vi "BigIntDevide.vi"(2 "b":cluster{"Boolean":bool, "Array":u64[]}, 3 "a":cluster{"Boolean":bool, "Array":u64[]}) -> (0 "a % b":cluster{"Boolean":bool, "Array":u64[]}, 1 "a / b":cluster{"Boolean":bool, "Array":u64[]})   [LabVIEW 2023]
panel:
  out "|b|":cluster{bool, "Array":u64[]}
  out "|a|":cluster{bool, "Array":u64[]}
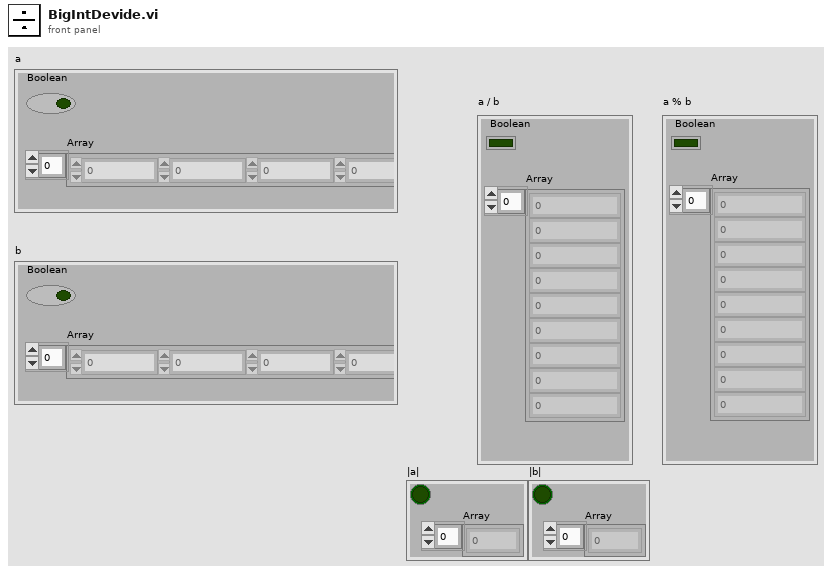
[diagram p1: front panel]
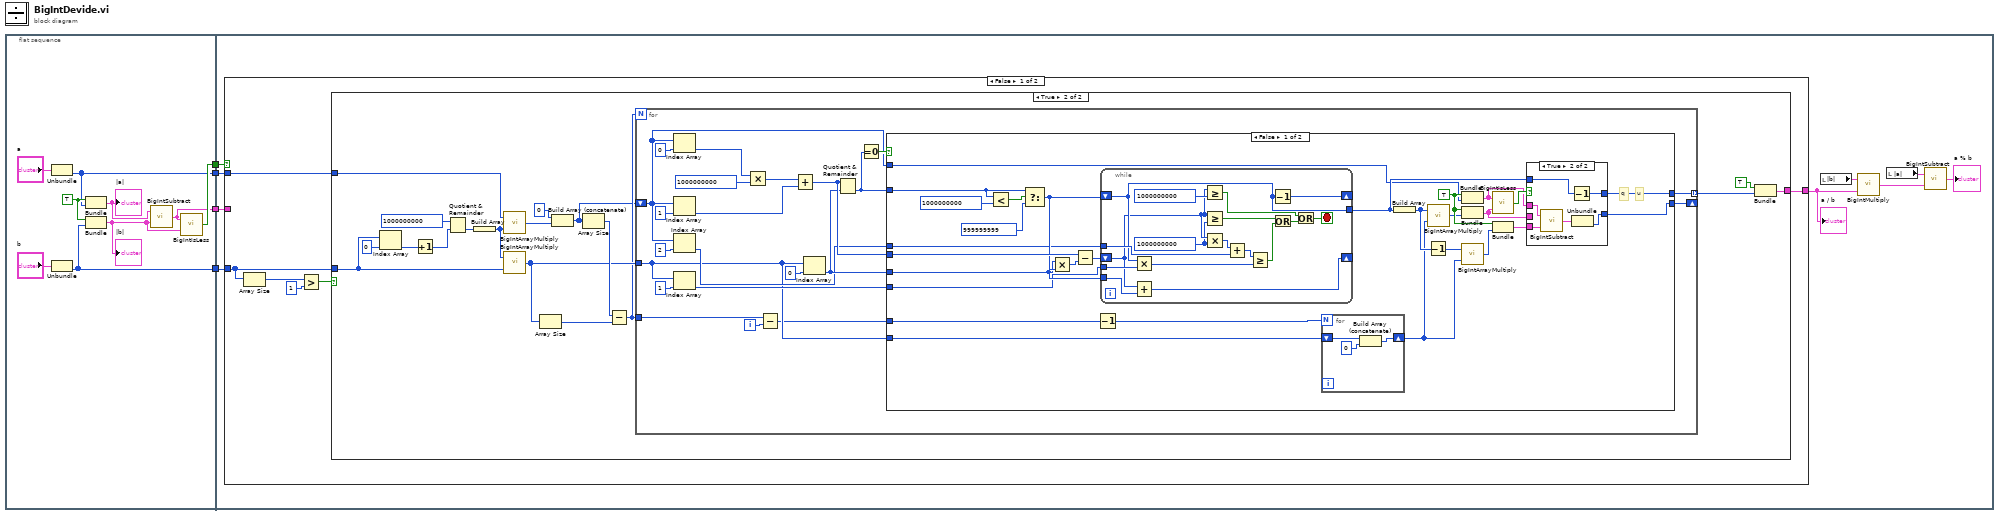
[diagram p0: block diagram]
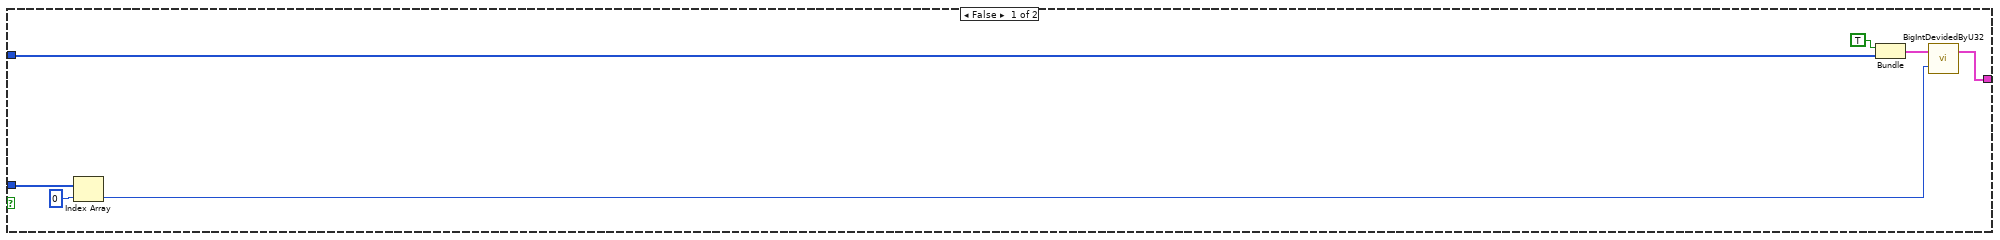
[diagram p2: hidden frame]
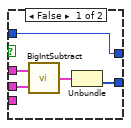
[diagram p3: hidden frame]
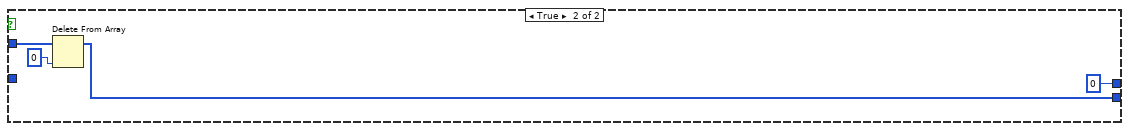
[diagram p4: hidden frame]
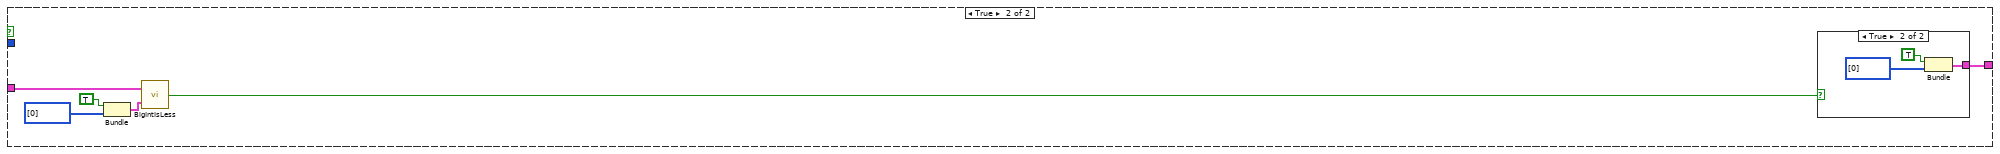
[diagram p5: hidden frame]
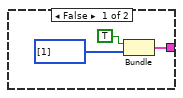
[diagram p6: hidden frame]
diagram:
  n1 = flat-sequence {
    tunnel: [w5] -> w4
    tunnel: [w6] -> w3
    tunnel: [w8] -> w2
    tunnel: [w7] -> w1
    tunnel: w4 -> [w17]
    tunnel: w3 -> [w16]
    tunnel: w2 -> [w15]
    tunnel: w1 -> [w14]
    frame #0 {
      w9 = TRUE
      n2 = Unbundle("a") -> ("Array"=w5:u64[])  [unwired: 1 out]
      n3 = Unbundle("b") -> ("Array"=w6:u64[])  [unwired: 1 out]
      n4 = Bundle(w9, "Array"=w5) -> (w12:cluster{bool, "Array":u64[]})  [unwired: 1 in]
      "|a|" <- w12
      n5 = Bundle(w9, "Array"=w6) -> (w13:cluster{bool, "Array":u64[]})  [unwired: 1 in]
      "|b|" <- w13
      n6 = call "BigIntSubtract.vi"("b"=w13, "a"=w12) -> ("a - b"=w7:cluster{"Boolean":bool, "Array":u64[]})
      n7 = call "BigIntIsLess.vi"("b"=w13, "a"=w7) -> ("a < b"=w8:bool)
    }
    frame #1 {
      n8 = case shown="False" w15 {
        tunnel: [w28 w139] -> w22
        tunnel: w17 -> [w27 _]
        tunnel: w16 -> [w26 _]
        tunnel: w14 -> [_ w142]
        frame False {
          n9 = Array Size(array=w26) -> (size(s)=w25:i32)
          n10 = Greater?(x=w25, y=1) -> (0:w23:bool)
          n11 = case shown="True" w23 {
            tunnel: [w29 w40] -> w28
            tunnel: w27 -> [w34 w39]
            tunnel: w26 -> [w33 w38]
            frame False {
              n12 = Index Array(array=w33, index=0) -> (element=w30:u64)
              n13 = Bundle(TRUE, "Array"=w34) -> (w31:cluster{bool, "Array":u64[]})  [unwired: 1 in]
              n14 = call "BigIntDevidedByU32.vi"("b (<1e9)"=w30, "a"=w31) -> ("a / b"=w29:cluster{"Boolean":bool, "Array":u64[]})  [unwired: 1 out]
            }
            frame True {
              n15 = Index Array(array=w38, index=0) -> (element=w52:u64)
              n16 = Increment(x=w52) -> (x+1=w51:u64)
              n17 = Quotient & Remainder(x=u64 1000000000, y=w51) -> (floor(x/y)=w49:u64)  [unwired: 1 out]
              n18 = Build Array(w49) -> (w48:u64[])
              n19 = call "BigIntArrayMultiply.vi"("b"=w48, "a"=w39) -> ("a * b"=w45:u64[])
              n20 = call "BigIntArrayMultiply.vi"("b"=w38, "a"=w48) -> ("a * b"=w44:u64[])
              n21 = Array Size(array=w44) -> (size(s)=w46:i32)
              n22 = Build Array (concatenate)(u64 0, w45) -> (w37:u64[])
              n23 = Array Size(array=w37) -> (size(s)=w47:i32)
              n24 = Subtract(x=w47, y=w46) -> (x-y=w43:i32)
              n25 = for {
                N: w43 -> [_]
                tunnel: w44 -> [w66]
                shift-right: [w60] -> _
                shift-left: w37 -> [w58]
                tunnel: w43 -> [w63]
                tunnel: [w61] -> w42 mode=indexing
                i -> [w57]
                n26 = Index Array(array=w58, index=0) -> (element=w59:u64)
                n27 = Index Array(array=w58, index=1) -> (element=w74:u64)
                n28 = Index Array(array=w58, index=2) -> (element=w67:u64)
                n29 = Index Array(array=w66, index=1) -> (element=w68:u64)
                n30 = Multiply(x=w59, y=u64 1000000000) -> (x*y=w65:u64)
                n31 = Subtract(x=w63, y=w57) -> (x-y=w62:i32)
                n32 = Add(x=w65, y=w74) -> (x+y=w71:u64)
                n33 = Index Array(array=w66, index=0) -> (element=w70:u64)
                n34 = Quotient & Remainder(x=w71, y=w70) -> (floor(x/y)=w72:u64)  [unwired: 1 out]
                n35 = Equal To 0?(x=w72) -> (x = 0?=w73:bool)
                n36 = case shown="False" w73 {
                  tunnel: w72 -> [w101 _]
                  tunnel: w71 -> [w99 _]
                  tunnel: w70 -> [w95 _]
                  tunnel: w68 -> [w94 _]
                  tunnel: w67 -> [w93 _]
                  tunnel: w58 -> [w83 w138]
                  tunnel: w66 -> [w92 _]
                  tunnel: w62 -> [w91 _]
                  tunnel: [w86 0] -> w61
                  tunnel: [w76 w136] -> w60
                  frame False {
                    w84 = TRUE
                    # "u"
                    # "q"
                    n37 = Less?(x=w101, y=u64 1000000000) -> (x < y?=w102:bool)
                    n38 = Select(t=w101, s=w102, f=u64 999999999) -> (s? t:f=w96:u64)
                    n39 = Multiply(x=w95, y=w96) -> (x*y=w98:u64)
                    n40 = Subtract(x=w99, y=w98) -> (x-y=w97:u64)
                    n41 = Decrement(x=w91) -> (x-1=w85:i32)
                    n42 = while {
                      tunnel: w95 -> [w133]
                      tunnel: w94 -> [w134]
                      shift-right: [w132] -> _
                      shift-left: w97 -> [w122]
                      shift-right: [w131] -> _
                      shift-left: w96 -> [w126]
                      tunnel: w93 -> [w129]
                      tunnel: [w126] -> w87
                      stop <- w123 stop-if-true
                      w121 = u64 1000000000
                      n43 = Multiply(x=w126, y=w134) -> (x*y=w127:u64)
                      n44 = Add(x=w122, y=w133) -> (x+y=w132:u64)
                      n45 = Greater Or Equal?(x=w122, y=u64 1000000000) -> (x >= y?=w124:bool)
                      n46 = Greater Or Equal?(x=w122, y=w121) -> (x >= y?=w120:bool)
                      n47 = Multiply(x=w122, y=w121) -> (x*y=w130:u64)
                      n48 = Add(x=w130, y=w129) -> (x+y=w128:u64)
                      n49 = Greater Or Equal?(x=w128, y=w127) -> (x >= y?=w119:bool)
                      n50 = Decrement(x=w126) -> (x-1=w131:u64)
                      n51 = Or(x=w120, y=w119) -> (x .or. y?=w118:bool)
                      n52 = Or(x=w124, y=w118) -> (x .or. y?=w123:bool)
                    }
                    n53 = for {
                      N: w85 -> [_]
                      shift-right: [w115] -> w89
                      shift-left: w92 -> [w117]
                      n54 = Build Array (concatenate)(w117, u64 0) -> (w115:u64[])
                    }
                    n55 = Build Array(w87) -> (w90:u64[])
                    n56 = Decrement(x=w90) -> (x-1=w88:u64[])
                    n57 = call "BigIntArrayMultiply.vi"("b"=w89, "a"=w90) -> ("a * b"=w82:u64[])
                    n58 = Bundle(w84, w83) -> (w79:cluster{bool, u64[]})  [unwired: 1 in]
                    n59 = Bundle(w84, "a * b"=w82) -> (w78:cluster{bool, "a * b":u64[]})  [unwired: 1 in]
                    n60 = call "BigIntArrayMultiply.vi"("b"=w89, "a"=w88) -> ("a * b"=w81:u64[])
                    n61 = call "BigIntIsLess.vi"("b"=w78, "a"=w79) -> ("a < b"=w80:bool)
                    n62 = Bundle(w84, "a * b"=w81) -> (w77:cluster{bool, "a * b":u64[]})  [unwired: 1 in]
                    n63 = case shown="True" w80 {
                      tunnel: w87 -> [w108 w114]
                      tunnel: [w108 w113] -> w86
                      tunnel: w79 -> [w107 w110]
                      tunnel: w78 -> [w106 _]
                      tunnel: w77 -> [_ w111]
                      tunnel: [w104 w109] -> w76
                      frame False {
                        n64 = call "BigIntSubtract.vi"("b"=w106, "a"=w107) -> ("a - b"=w105:cluster{"Boolean":bool, "Array":u64[]})
                        n65 = Unbundle(w105) -> ("Array"=w104:u64[])  [unwired: 1 out]
                      }
                      frame True {
                        n66 = call "BigIntSubtract.vi"("b"=w111, "a"=w110) -> ("a - b"=w112:cluster{"Boolean":bool, "Array":u64[]})
                        n67 = Decrement(x=w114) -> (x-1=w113:u64)
                        n68 = Unbundle(w112) -> ("Array"=w109:u64[])  [unwired: 1 out]
                      }
                    }
                  }
                  frame True {
                    n69 = Delete From Array(array=w138, index=0) -> (array with subset deleted=w136:u64[])  [unwired: 1 in, 1 out]
                  }
                }
              }
              n70 = Bundle(TRUE, w42) -> (w40:cluster{bool, u64[]})  [unwired: 1 in]
            }
          }
        }
        frame True {
          n71 = Bundle(TRUE, u64[] [0]) -> (w141:cluster{bool, u64[]})  [unwired: 1 in]
          n72 = call "BigIntIsLess.vi"("b"=w141, "a"=w142) -> ("a < b"=w140:bool)
          n73 = case shown="True" w140 {
            tunnel: [w145 w148] -> w139
            frame False {
              n74 = Bundle(TRUE, u64[] [1]) -> (w145:cluster{bool, u64[]})  [unwired: 1 in]
            }
            frame True {
              n75 = Bundle(TRUE, u64[] [0]) -> (w148:cluster{bool, u64[]})  [unwired: 1 in]
            }
          }
        }
      }
      "a / b" <- w22
      n76 = local read "|b|"() -> (w19:cluster{bool, "Array":u64[]})
      n77 = call "BigIntMultiply.vi"("b"=w22, "a"=w19) -> ("a * b"=w21:cluster{"Boolean":bool, "Array":u64[]})
      n78 = local read "|a|"() -> (w18:cluster{bool, "Array":u64[]})
      n79 = call "BigIntSubtract.vi"("b"=w21, "a"=w18) -> ("a - b"=→"a % b":cluster{"Boolean":bool, "Array":u64[]})
    }
  }
